vi "Initialize.vi"(8 "error in (no error)":errorcluster, 9 "Reset (True)":bool=TRUE, 10 "ID Query (True)":bool=TRUE, 11 "VISA resource name":refnum<visa-resource-name>) -> (0 "error out":errorcluster, 3 "VISA resource name out":refnum<visa-resource-name>)   [LabVIEW 2018, in "Keithley KE22xx Series.lvlib"]
doc: "Establishes communication with the instrument and optionally performs an instrument identification query and/or an instrument reset. It also places the instrument in a default state needed for other instrument driver operations. Therefore, call this VI before calling other instrument driver VIs for this instrument. Generally, you need to call the Initialize VI only once at the beginning of an application."
uses:
  Keithley KE22xx Series.lvlib
  <vilib>/Instr/_visa.llb/VISA Configure Serial Port (Instr).vi
panel:
  # "© 2012 Keithley Instruments, Inc. ALL RIGHTS RESERVED"
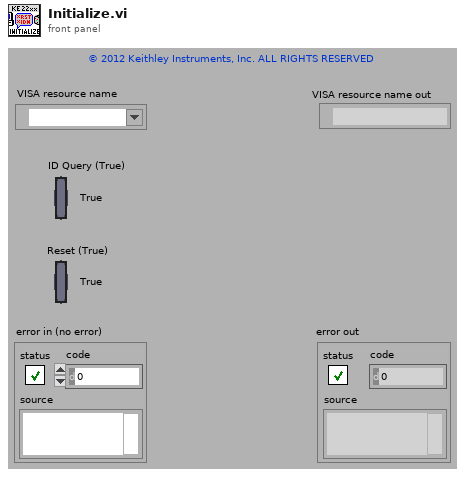
[diagram p1: front panel]
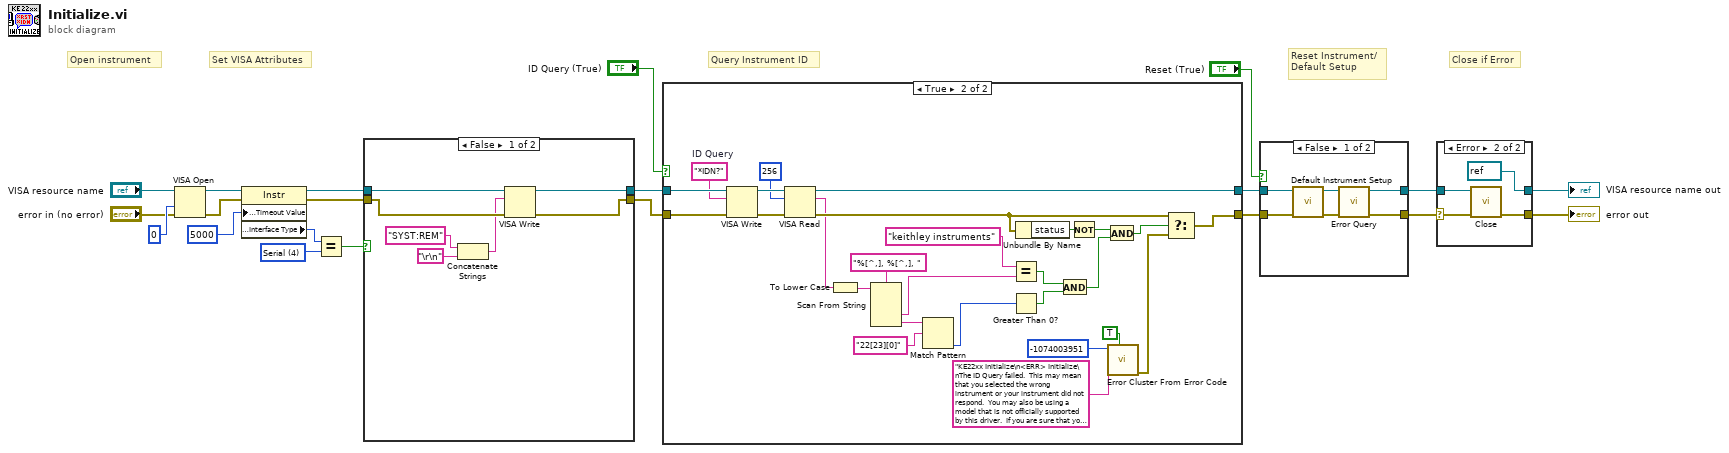
[diagram p0: block diagram]
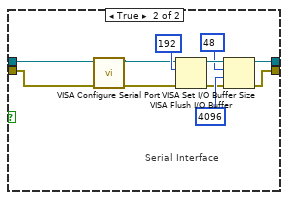
[diagram p2: hidden frame]
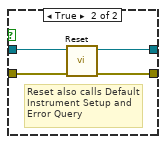
[diagram p4: hidden frame]
diagram:
  w10 = u16 4 items=["GPIB"=1, "VXI"=2, "GPIB-VXI"=3, "Serial"=4, "PXI"=5, "TCPIP"=6, "USB"=7] ("Interface Information:Interface Type")
  # "Set VISA Attributes"
  # "Close if Error"
  # "Query Instrument ID"
  # "Reset Instrument/\nDefault Setup"
  # "Open instrument"
  n1 = VISA Open(access mode=u32 0, error in (no error)="error in (no error)", VISA resource name="VISA resource name") -> (VISA resource name=w4:refnum<visa-resource-name>, error out=w3:errorcluster)  [unwired: 2 in]
  n2 = property class="Instr"(reference=w4, error in=w3, "General Settings:Timeout Value"=u32 5000) -> (reference out=w13:refnum<visa-resource-name>, error out=w12:errorcluster, "Interface Information:Interface Type"=w17:u16)
  n3 = Equal?(x=w17, y=w10) -> (x = y?=w11:bool)
  n4 = case shown="False" w11 {
    tunnel: [w27 w32] -> w15
    tunnel: [w25 w29] -> w14
    tunnel: w13 -> [w28 w31]
    tunnel: w12 -> [w26 w30]
    frame False {
      n5 = Concatenate Strings("SYST:REM", "\r\n") -> (w22:string)
      n6 = VISA Write(VISA resource name=w28, write buffer=w22, error in (no error)=w26) -> (VISA resource name out=w27:refnum<visa-resource-name>, error out=w25:errorcluster)  [unwired: 1 out]
    }
    frame True {
      # "Serial Interface"
      n7 = call-poly "VISA Configure Serial Port"("VISA resource name"=w31, "error in (no error)"=w30) -> ("VISA resource name out"=w33:refnum<visa-resource-name>, "error out"=w34:errorcluster)  [unwired: 4 in, 8 out]
      n8 = VISA Flush I/O Buffer(VISA resource name=w33, mask (16)=u16 192, error in (no error)=w34) -> (VISA resource name out=w37:refnum<visa-resource-name>, error out=w38:errorcluster)
      n9 = VISA Set I/O Buffer Size(VISA resource name=w37, mask (16)=u16 48, size (4096)=u32 4096, error in (no error)=w38) -> (VISA resource name out=w32:refnum<visa-resource-name>, error out=w29:errorcluster)
    }
  }
  n10 = case shown="True" "ID Query (True)" {
    tunnel: [w40 w68] -> w20
    tunnel: [w41 w65] -> w21
    tunnel: w15 -> [w41 w66]
    tunnel: w14 -> [w40 w67]
    frame False {
    }
    frame True {
      w61 = "*IDN?"  # ID Query
      n11 = VISA Write(VISA resource name=w66, write buffer=w61, error in (no error)=w67) -> (VISA resource name out=w64:refnum<visa-resource-name>, error out=w63:errorcluster)  [unwired: 1 out]
      n12 = VISA Read(VISA resource name=w64, byte count=u32 256, error in (no error)=w63) -> (VISA resource name out=w65:refnum<visa-resource-name>, read buffer=w42:string, error out=w43:errorcluster)  [unwired: 1 out]
      n13 = To Lower Case(string=w42) -> (all lower case string=w51:string)
      n14 = Scan From String(format string="%[^,], %[^,], ", input string=w51) -> (output 1=w53:string, output 2=w55:string)  [unwired: 2 in, 5 out]
      n15 = Match Pattern(string=w55, regular expression="22[23][0]") -> (offset past match=w47:i32)  [unwired: 4 out]
      n16 = Equal?(x="keithley instruments" ("regular expression"), y=w53) -> (x = y?=w54:bool)
      n17 = Greater Than 0?(x=w47) -> (x > 0?=w48:bool)
      n18 = Unbundle By Name(w43) -> ("status"=w45:bool)
      n19 = And(x=w54, y=w48) -> (x .and. y?=w49:bool)
      n20 = Not(x=w45) -> (.not. x?=w56:bool)
      n21 = And(x=w56, y=w49) -> (x .and. y?=w44:bool)
      n22 = call <vilib>:"Error Cluster From Error Code.vi"("show call chain? (False)"=TRUE, "error message (\"\")"="KE22xx Initialize\n<ERR> Initialize\nThe ID Query failed.  This may mean that you selected the wrong instrument or your instrument did not respond.  You may also be using a model that is not officially supported by this driver.  If you are sure that you have selected the correct instrument and it is responding, try disabling the ID Query." ("Source (VI Name)"), "error code (0)"=-1074003951) -> ("error out"=w60:errorcluster)  [unwired: 6 in]
      n23 = Select(t=w43, s=w44, f=w60) -> (s? t:f=w68:errorcluster)
    }
  }
  n24 = case shown="False" "Reset (True)" {
    tunnel: w20 -> [w73 w75]
    tunnel: [w70 w78] -> w5
    tunnel: w21 -> [w74 w76]
    tunnel: [w71 w77] -> w6
    frame False {
      n25 = call "Default Instrument Setup.vi"("error in (no error)"=w73, "VISA resource name"=w74) -> ("error out"=w69:errorcluster, "VISA resource name out"=w72:refnum<visa-resource-name>)  [unwired: 8 in]
      n26 = call "Error Query.vi"("error in (no error)"=w69, "VISA resource name"=w72) -> ("error out"=w70:errorcluster, "VISA resource name out"=w71:refnum<visa-resource-name>)  [unwired: 6 in, 2 out]
    }
    frame True {
      # "Reset also calls Default Instrument Setup and Error Query"
      n27 = call "Reset.vi"("error in (no error)"=w75, "VISA resource name"=w76) -> ("error out"=w78:errorcluster, "VISA resource name out"=w77:refnum<visa-resource-name>)  [unwired: 8 in]
    }
  }
  n28 = case shown="Error" w5 {
    selector: w5 -> [w79 w82]
    tunnel: w6 -> [w80 w83]
    tunnel: [w80 refnum<visa-resource-name> refnum ("VISA resource name out")] -> w8
    tunnel: [w79 w84] -> w7
    frame No Error {
    }
    frame Error {
      n29 = call "Close.vi"("error in (no error)"=w82, "VISA resource name"=w83) -> ("error out"=w84:errorcluster)  [unwired: 9 in]
    }
  }
  "VISA resource name out" <- w8
  "error out" <- w7
